vi "2283_autoAlign.vi"() -> (0 "output":dbl format="%.2f")   [LabVIEW 2014]
uses:
  <vilib>/Rock Robotics/Network Tables/SD Read Number.vi
  <vilib>/addons/control/pid/pid.llb/PID (DBL).vi
  <vilib>/addons/control/pid/NI_PID_pid.lvlib
panel:
  in  "Numeric":dbl=0.1 format="%#_13g"
  in  "PID gains":T1={"proportional gain (Kc)"=1.8, "integral time (Ti, min)"=0.0, "derivative time (Td, min)"=0.0}
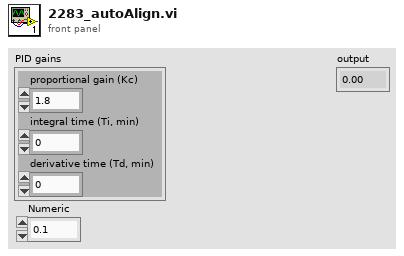
[diagram p1: front panel]
types:
  T1 = cluster{"proportional gain (Kc)":dbl, "integral time (Ti, min)":dbl, "derivative time (Td, min)":dbl}
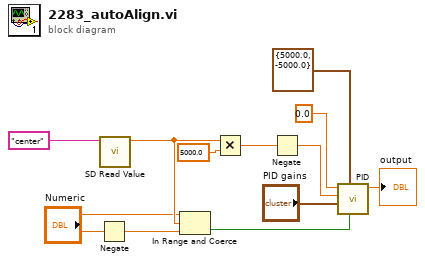
[diagram p0: block diagram]
diagram:
  n1 = Negate(x="Numeric") -> (-x=w2:dbl)
  n2 = call-poly <vilib>:"SD Read Value.vi"("Name"="center") -> ("Numeric"=w4:dbl)  [unwired: 8 in, 2 out]
  n3 = In Range and Coerce(upper limit="Numeric", x=w4, lower limit=w2) -> (In Range?=w1:bool)  [unwired: 1 out]
  n4 = Multiply(x=w4, y=5000.0) -> (x*y=w7:dbl)
  n5 = Negate(x=w7) -> (-x=w6:dbl)
  n6 = call-poly <vilib>:"PID.vi"("reinitialize? (F)"=w1, "output range"=cluster{"output high":dbl, "output low":dbl} {"output high"=5000.0, "output low"=-5000.0}, "PID gains"="PID gains", "process variable"=w6, "setpoint"=0.0) -> ("output"=→"output":dbl)  [unwired: 5 in, 1 out]
